vi "_LoadMolanaMethod.vi"(7 "HasESI2":bool, 8 "HasESI1":bool=TRUE, 9 "Path":path=path "C:/Users/Public/Instrument/Project-Service/MS Methods/Automated Calibration Methods/Q1 PPG POS Default.method") -> (0 "error out":errorcluster, 1 "MethodLevelParameters":string[][](array[string]), 2 "Expt":string[](array[string]), 3 "Method":string[](array[string]), 4 "UseESI1":bool, 5 "ExptParamAndMR":T2)   [LabVIEW 2015]
uses:
  Type/_Mass Range Parameters.ctl
  Type/_Log Command.ctl
  Controls/xml Parameter Type.ctl
  <vilib>/xml/Close Reference(Node).vi
  <vilib>/xml/Close Reference(NNMap).vi
  <resource>/objmgr/DOMUserDefRef.rc
  <vilib>/xml/NI_XML.lvlib
panel:
  in  "error in (no error)":errorcluster
  # "APCI1             APCI2               ESI1                ESI2              Expt#              Eq                 Scan#"
  # "Num             Type            Polarity        StartTime      StopTime        Cycles       PauseTime    DelayTime          MR#         DwellTime   Comment"
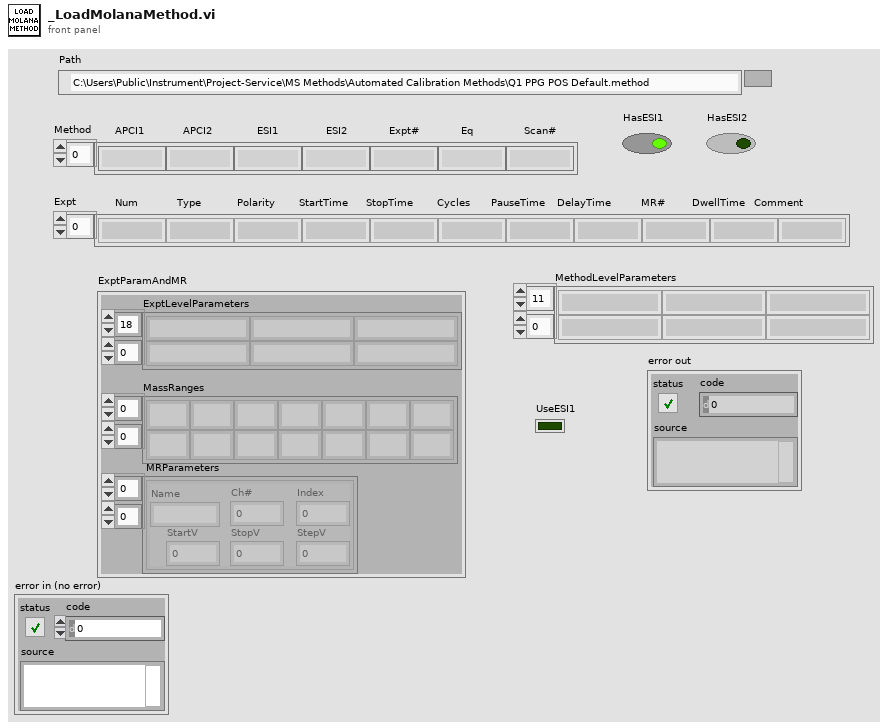
[diagram p1: front panel]
types:
  T1 = typedef "_Mass Range Parameters.ctl" = cluster{"Name":string, "Ch#":u8, "StartV":dbl, "StopV":dbl, "StepV":dbl, "Index":u8}
  T2 = cluster{"ExptLevelParameters":string[][], "MassRanges":string[][], " MRParameters":T1[][]}
  T3 = typedef "_Log Command.ctl" = enum16{"No Command", "Open", "Read", "Write", "Close", "Check Size"}
  T4 = typedef "xml Parameter Type.ctl" = enum16{"Method Parameters", "Experiment Parameters"}
  T5 = cluster{"ExptLevelParameters":string[][], "MassRanges":string[][], " MRParameters":T1[][]}[]
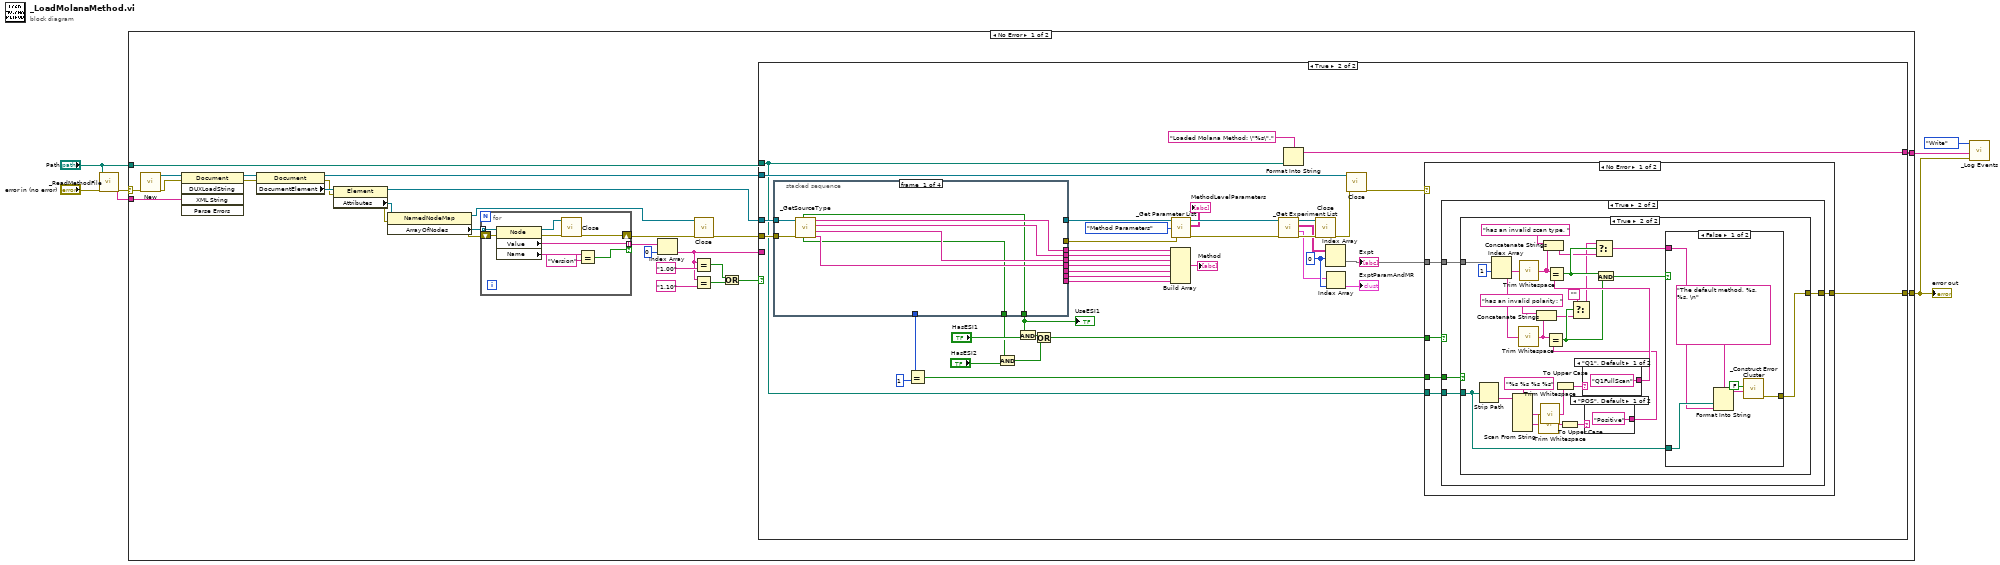
[diagram p0: block diagram]
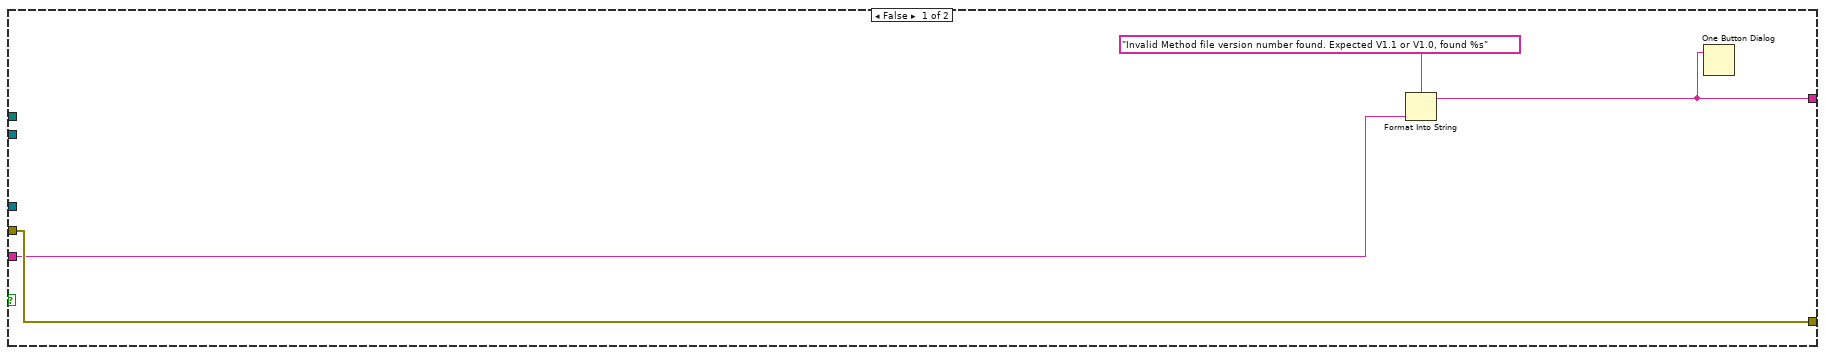
[diagram p2: hidden frame]
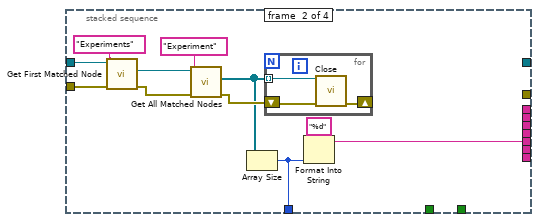
[diagram p3: hidden frame]
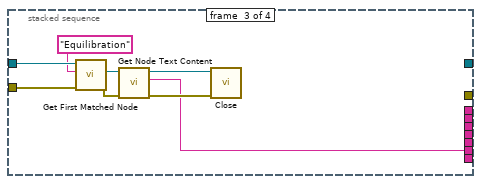
[diagram p4: hidden frame]
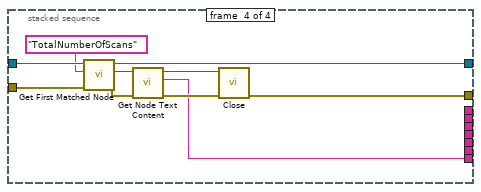
[diagram p5: hidden frame]
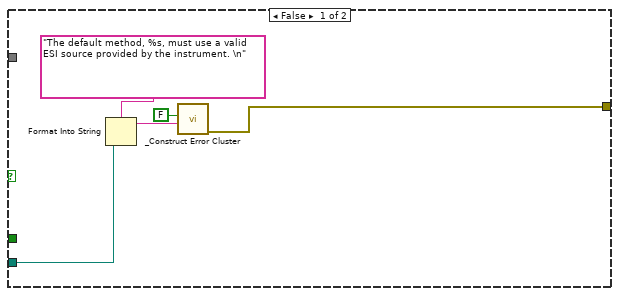
[diagram p6: hidden frame]
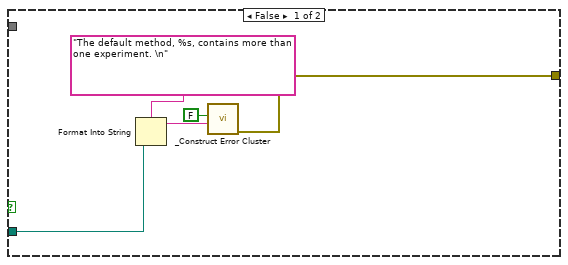
[diagram p7: hidden frame]
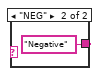
[diagram p9: hidden frame]
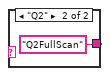
[diagram p10: hidden frame]
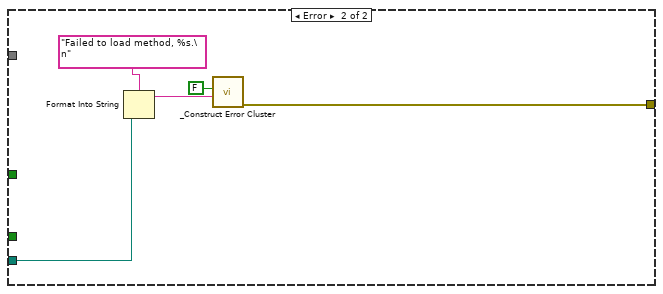
[diagram p11: hidden frame]
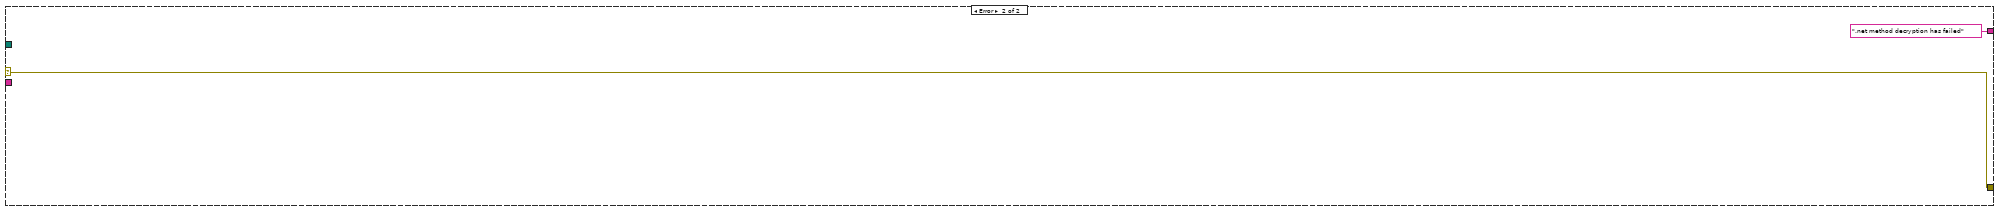
[diagram p12: hidden frame]
diagram:
  n1 = call "_ReadMethodFile.vi"("error in (no error)"="error in (no error)", "Path"="Path") -> ("error out"=w4:errorcluster, "LVGetMethodXML"=w1:string)  [unwired: 8 in]
  n2 = case shown="No Error" w4 {
    selector: w4 -> [w14 w192]
    tunnel: [w24 w192] -> w6
    tunnel: [w23 ".net method decryption has failed"] -> w5
    tunnel: "Path" -> [w9 _]
    tunnel: w1 -> [w8 _]
    frame No Error {
      n3 = call <vilib>:"New.vi"("error in (no error)"=w14) -> ("error out"=w12:errorcluster, "DOM document out"=w13:refnum<k20>)  [unwired: 7 in]
      n4 = invoke class="Document" method="DUXLoadString"(reference=w13, error in=w12, "XML String"=w8) -> (reference out=w10:refnum<k20>, error out=w11:errorcluster)  [unwired: 2 in, 3 out]
      n5 = property on="Property Node" class="Document"(reference=w10, error in=w11) -> (reference out=w35:refnum<k20>, error out=w30:errorcluster, "DocumentElement"=w32:refnum<k20>)
      n6 = property on="Property Node" class="Element"(reference=w32, error in=w30) -> (reference out=w31:refnum<k20>, error out=w29:errorcluster, "Attributes"=w34:refnum<k20>)
      n7 = property on="Property Node" class="NamedNodeMap"(reference=w34, error in=w29) -> (reference out=w25:refnum<k20>, error out=w28:errorcluster, "ArrayOfNodes"=w33:refnum<k20>[])
      n8 = for {
        tunnel: w33 -> [w190] mode=indexing
        shift-right: [w184] -> w27
        shift-left: w28 -> [w189]
        tunnel: [w183] -> w18 mode=indexing if=w182
        n9 = property on="Property Node" class="Node"(reference=w190, error in=w189) -> (reference out=w185:refnum<k20>, error out=w186:errorcluster, "Value"=w183:string, "Name"=w187:string)
        n10 = call-poly <vilib>:"Close.vi"("error in (no error)"=w186, "node"=w185) -> ("error out"=w184:errorcluster)  [unwired: 7 in]
        n11 = Equal?(x=w187, y="Version" ("x")) -> (x = y?=w182:bool)
      }
      n12 = Index Array(array=w18, index=0) -> (element=w15:string)
      n13 = call-poly <vilib>:"Close.vi"("error in (no error)"=w27, "named node map"=w25) -> ("error out"=w26:errorcluster)  [unwired: 7 in]
      n14 = Equal?(x=w15, y="1.00") -> (x = y?=w20:bool)
      n15 = Equal?(x=w15, y="1.10") -> (x = y?=w22:bool)
      n16 = Or(x=w20, y=w22) -> (x .or. y?=w16:bool)
      n17 = case shown="True" w16 {
        tunnel: w35 -> [_ w79]
        tunnel: w31 -> [_ w60]
        tunnel: w26 -> [w39 w59]
        tunnel: w9 -> [_ w49]
        tunnel: [w39 w41] -> w24
        tunnel: [w36 w40] -> w23
        tunnel: w15 -> [w37 _]
        frame False {
          n18 = Format Into String(format string="Invalid Method file version number found. Expected V1.1 or V1.0, found %s", w37) -> (resulting string=w36:string)  [unwired: 2 in, 1 out]
          n19 = One Button Dialog(message=w36) -> ()  [unwired: 1 in, 1 out]
        }
        frame True {
          w62 = 0 ("index (row)")
          n20 = stacked-sequence {
            tunnel: w60 -> [w87 w98 w109 w119]
            tunnel: w59 -> [w80 w97 w108 w118]
            tunnel: [w86 _ _ _] -> w72
            tunnel: [w85 _ _ _] -> w73
            tunnel: [w84 _ _ _] -> w74
            tunnel: [w83 _ _ _] -> w75
            tunnel: [_ w96 _ _] -> w76
            tunnel: [_ _ w102 _] -> w77
            tunnel: [_ _ _ w112] -> w78
            tunnel: [_ _ _ w111] -> w68
            tunnel: [_ _ _ w110] -> w67
            tunnel: [w81 _ _ _] -> w44
            tunnel: [w82 _ _ _] -> w55
            tunnel: [_ w95 _ _] -> w48
            frame #0 {
              n21 = call "_GetSourceType.vi"("error in (no error)"=w80, "node in"=w87) -> ("ESI2"=w83:string, "ESI1"=w84:string, "APCI2"=w85:string, "APCI1"=w86:string, "HasESI2"=w82:bool, "HasESI1"=w81:bool)  [unwired: 2 in]
            }
            frame #1 {
              n22 = call <vilib>:"Get First Matched Node.vi"("error in (no error)"=w97, "XPath expression"="Experiments", "node in"=w98) -> ("error out"=w92:errorcluster, "node result"=w93:refnum<k20>)  [unwired: 6 in, 1 out]
              n23 = call <vilib>:"Get All Matched Nodes.vi"("error in (no error)"=w92, "XPath expression"="Experiment", "node in"=w93) -> ("error out"=w91:errorcluster, "node result array"=w90:refnum<k20>[])  [unwired: 6 in, 1 out]
              n24 = Array Size(array=w90) -> (size(s)=w95:i32)
              n25 = for {
                tunnel: w90 -> [w101] mode=indexing
                shift-right: [w99] -> _
                shift-left: w91 -> [w100]
                n26 = call-poly <vilib>:"Close.vi"("error in (no error)"=w100, "node"=w101) -> ("error out"=w99:errorcluster)  [unwired: 7 in]
              }
              n27 = Format Into String(format string="%d", w95) -> (resulting string=w96:string)  [unwired: 2 in, 1 out]
            }
            frame #2 {
              n28 = call <vilib>:"Get First Matched Node.vi"("error in (no error)"=w108, "XPath expression"="Equilibration", "node in"=w109) -> ("error out"=w104:errorcluster, "node result"=w106:refnum<k20>)  [unwired: 6 in, 1 out]
              n29 = call <vilib>:"Get Node Text Content.vi"("error in (no error)"=w104, "node in"=w106) -> ("error out"=w103:errorcluster, "node text"=w102:string, "node out"=w105:refnum<k20>)  [unwired: 7 in]
              n30 = call-poly <vilib>:"Close.vi"("error in (no error)"=w103, "node"=w105) -> ()  [unwired: 7 in, 1 out]
            }
            frame #3 {
              n31 = call <vilib>:"Get First Matched Node.vi"("error in (no error)"=w118, "XPath expression"="TotalNumberOfScans", "node in"=w119) -> ("error out"=w115:errorcluster, "node result"=w116:refnum<k20>, "node out"=w111:refnum<k20>)  [unwired: 6 in]
              n32 = call <vilib>:"Get Node Text Content.vi"("error in (no error)"=w115, "node in"=w116) -> ("error out"=w114:errorcluster, "node text"=w112:string, "node out"=w113:refnum<k20>)  [unwired: 7 in]
              n33 = call-poly <vilib>:"Close.vi"("error in (no error)"=w114, "node"=w113) -> ("error out"=w110:errorcluster)  [unwired: 7 in]
            }
          }
          "UseESI1" <- w44
          n34 = Equal?(x=w48, y=1) -> (x = y?=w46:bool)
          n35 = And(x=w55, y="HasESI2") -> (x .and. y?=w53:bool)
          n36 = And(x=w44, y="HasESI1") -> (x .and. y?=w52:bool)
          n37 = Or(x=w52, y=w53) -> (x .or. y?=w50:bool)
          n38 = Build Array(w72, w73, w74, w75, w76, w77, w78) -> (→"Method":string[])
          n39 = call "_Get Parameter List.vi"("error in (no error)"=w67, "Parameter Type"=xml_Parameter_Type."Method Parameters", "node in"=w68) -> ("error out"=w70:errorcluster, "Parameters List"=→"MethodLevelParameters":string[][], "node out"=w69:refnum<k20>)  [unwired: 2 in]
          n40 = call "_Get Experiment List.vi"("error in (no error)"=w70, "node in"=w69) -> ("error out"=w64:errorcluster, "ExptParamAndMR"=w43:T5, "Expt"=w63:string[][], "node out"=w65:refnum<k20>)  [unwired: 2 in]
          n41 = Format Into String(format string="Loaded Molana Method: \"%s\".", w49) -> (resulting string=w40:string)  [unwired: 2 in, 1 out]
          n42 = call-poly <vilib>:"Close.vi"("error in (no error)"=w64, "node"=w65) -> ("error out"=w58:errorcluster)  [unwired: 7 in]
          n43 = Index Array(array=w63, index (row)=w62) -> (element=w45:string[])  [unwired: 1 in]
          "Expt" <- w45
          n44 = Index Array(array=w43, index=w62) -> (element=→"ExptParamAndMR":T2)
          n45 = call-poly <vilib>:"Close.vi"("error in (no error)"=w58, "node"=w79) -> ("error out"=w51:errorcluster)  [unwired: 7 in]
          n46 = case shown="No Error" w51 {
            tunnel: w50 -> [w124 _]
            tunnel: w49 -> [w122 w179]
            tunnel: [w123 w178] -> w41
            tunnel: w46 -> [w121 _]
            tunnel: w45 -> [w120 _]
            frame No Error {
              n47 = case shown="True" w124 {
                tunnel: [w127 w131] -> w123
                tunnel: w122 -> [w126 w132]
                tunnel: w121 -> [_ w133]
                tunnel: w120 -> [_ w130]
                frame False {
                  n48 = Format Into String(format string="The default method, %s, must use a valid ESI source provided by the instrument. \n", w126) -> (resulting string=w128:string)  [unwired: 2 in, 1 out]
                  n49 = call "_Construct Error Cluster.vi"("reason"=w128, "CallingChain? (T)"=FALSE) -> ("error out"=w127:errorcluster)  [unwired: 5 in]
                }
                frame True {
                  n50 = case shown="True" w133 {
                    tunnel: w132 -> [w136 w151]
                    tunnel: [w135 w139] -> w131
                    tunnel: w130 -> [_ w166]
                    frame False {
                      n51 = Format Into String(format string="The default method, %s, contains more than one experiment. \n", w136) -> (resulting string=w137:string)  [unwired: 2 in, 1 out]
                      n52 = call "_Construct Error Cluster.vi"("reason"=w137, "CallingChain? (T)"=FALSE) -> ("error out"=w135:errorcluster)  [unwired: 5 in]
                    }
                    frame True {
                      n53 = Strip Path(path=w151) -> (name=w164:string)  [unwired: 1 out]
                      n54 = Index Array(array=w166, index #1=1 ("index")) -> (element #1=w160:string, element #2=w158:string)  [unwired: 1 in]
                      n55 = Scan From String(format string="%s %s %s %s", input string=w164) -> (output 1=w162:string, output 3=w157:string)  [unwired: 8 in, 3 out]
                      n56 = call <vilib>:"Trim Whitespace.vi"("string"=w158) -> ("trimmed string"=w143:string)  [unwired: 1 in]
                      n57 = call <vilib>:"Trim Whitespace.vi"("string"=w160) -> ("trimmed string"=w149:string)  [unwired: 1 in]
                      n58 = Concatenate Strings("has an invalid polarity: " ("string"), w143) -> (w144:string)
                      n59 = call <vilib>:"Trim Whitespace.vi"("string"=w157) -> ("trimmed string"=w156:string)  [unwired: 1 in]
                      n60 = call <vilib>:"Trim Whitespace.vi"("string"=w162) -> ("trimmed string"=w161:string)  [unwired: 1 in]
                      n61 = Concatenate Strings("has an invalid scan type, " ("string"), w149) -> (w147:string)
                      n62 = To Upper Case(1:w161) -> (0:w155:string)
                      n63 = To Upper Case(1:w156) -> (0:w154:string)
                      n64 = case shown="\"Q1\", Default" w155 {
                        tunnel: ["Q1FullScan" "Q2FullScan"] -> w159
                        frame "Q1", Default {
                        }
                        frame "Q2" {
                        }
                      }
                      n65 = Equal?(x=w149, y=w159) -> (x = y?=w150:bool)
                      n66 = case shown="\"POS\", Default" w154 {
                        tunnel: ["Positive" "Negative"] -> w153
                        frame "POS", Default {
                        }
                        frame "NEG" {
                        }
                      }
                      n67 = Equal?(x=w143, y=w153) -> (x = y?=w146:bool)
                      n68 = Select(t="", s=w146, f=w144) -> (s? t:f=w141:string)
                      n69 = Select(t=w141, s=w150, f=w147) -> (s? t:f=w140:string)
                      n70 = And(x=w150, y=w146) -> (x .and. y?=w152:bool)
                      n71 = case shown="False" w152 {
                        tunnel: w151 -> [w171 _]
                        tunnel: w140 -> [w169 _]
                        tunnel: [w168 _] -> w139
                        frame False {
                          n72 = Format Into String(format string="The default method, %s,  %s. \n", w171, w169) -> (resulting string=w172:string)  [unwired: 2 in, 1 out]
                          n73 = call "_Construct Error Cluster.vi"("reason"=w172, "CallingChain? (T)"=FALSE) -> ("error out"=w168:errorcluster)  [unwired: 5 in]
                        }
                        frame True {
                        }
                      }
                    }
                  }
                }
              }
            }
            frame Error {
              n74 = Format Into String(format string="Failed to load method, %s.\n", w179) -> (resulting string=w180:string)  [unwired: 2 in, 1 out]
              n75 = call "_Construct Error Cluster.vi"("reason"=w180, "CallingChain? (T)"=FALSE) -> ("error out"=w178:errorcluster)  [unwired: 5 in]
            }
          }
        }
      }
    }
    frame Error {
    }
  }
  "error out" <- w6
  n76 = call "_Log Events.vi"("error in (no error)"=w6, "Event"=w5, "Log Command"=_Log_Command."Write" ("File Command")) -> ()  [unwired: 5 in, 2 out]
